vi "Insert Menu Item with Hierarchy.vi"(4 "after item":string, 5 "menu tag":string, 6 "error in":errorcluster, 7 "item tag":string, 8 "item name":string, 9 "menu reference":refnum<k9>) -> (0 "error out":errorcluster, 1 "item tags out":string[](array[string]), 3 "menu reference out":refnum<k9>)   [LabVIEW 2025, in "XNode Support.lvlib"]
uses:
  XNode Support.lvlib
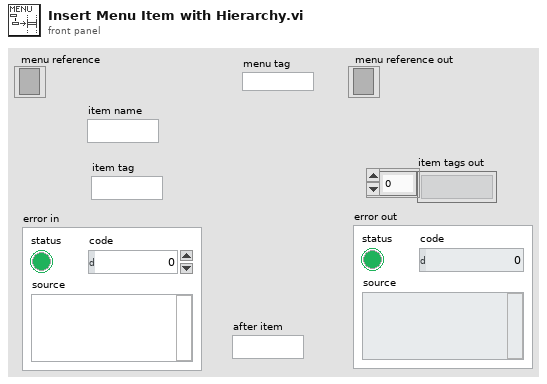
[diagram p1: front panel]
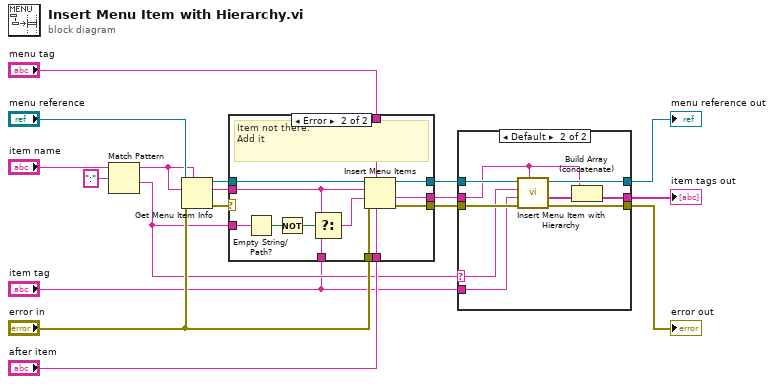
[diagram p0: block diagram]
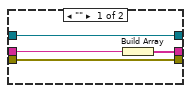
[diagram p3: hidden frame]
diagram:
  n1 = Match Pattern(string="item name", regular expression=":") -> (before substring=w4:string, after substring=w2:string)  [unwired: 1 in, 2 out]
  n2 = Get Menu Item Info(7:w4, 8:"error in", 11:"menu reference") -> (0:w3:errorcluster, 3:w5:refnum<k9>)  [unwired: 5 out]
  n3 = case shown="Error" w3 {
    selector: w3 -> [w18 _]
    tunnel: "menu tag" -> [_ w33]
    tunnel: "after item" -> [_ w32]
    tunnel: [w19 w31] -> w13
    tunnel: [w20 w30] -> w12
    tunnel: [w18 w29] -> w11
    tunnel: "error in" -> [_ w28]
    tunnel: w5 -> [w20 w27]
    tunnel: w4 -> [w19 w23]
    tunnel: w2 -> [_ w26]
    tunnel: "item tag" -> [_ w24]
    frame No Error {
      # "Already there"
    }
    frame Error {
      # "Item not there.\nAdd it"
      n4 = Empty String/Path?(string/path=w26) -> (empty?=w25:bool)
      n5 = Not(x=w25) -> (.not. x?=w21:bool)
      n6 = Select(t=w23, s=w21, f=w24) -> (s? t:f=w22:string)
      n7 = Insert Menu Items(4:w32, 5:w33, 6:w28, 7:w22, 8:w23, 9:w27) -> (0:w29:errorcluster, 1:w31:string, 3:w30:refnum<k9>)
    }
  }
  n8 = case shown="Default" w2 {
    selector: w2 -> [_ w44]
    tunnel: w13 -> [w37 w40]
    tunnel: w12 -> [w35 w46]
    tunnel: w11 -> [w34 w45]
    tunnel: [w35 w43] -> w10
    tunnel: [w36 w41] -> w9
    tunnel: [w34 w39] -> w8
    tunnel: "item tag" -> [_ w38]
    frame "" {
      n9 = Build Array(w37) -> (w36:string[])
    }
    frame Default {
      n10 = call "Insert Menu Item with Hierarchy.vi"("menu tag"=w40, "error in"=w45, "item tag"=w38, "item name"=w44, "menu reference"=w46) -> ("error out"=w39:errorcluster, "item tags out"=w42:string[], "menu reference out"=w43:refnum<k9>)  [unwired: 2 in]
      n11 = Build Array (concatenate)(w40, w42) -> (w41:string[])
    }
  }
  "menu reference out" <- w10
  "item tags out" <- w9
  "error out" <- w8
